vi "WriteHeader.vi"(2 "Filename":string, 3 "NXT":T1={"Hardware"="NXT", "Flattened String"=""}, 8 "File Size (2048)":u32=2048 caption="File Size (256)") -> (0 "NXT":T1={"Hardware"="NXT", "Flattened String"=""})   [LabVIEW 2010, in "Packet Recorder.lvlib"]
uses:
  Packet Recorder.lvlib
  <vilib>/NXT/Subs/LVHSConnector.ctl
  Components/Components.lvlib
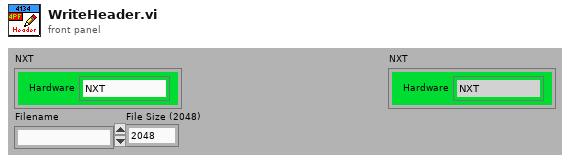
[diagram p1: front panel]
types:
  T1 = typedef "LVHSConnector.ctl" = cluster{"Hardware":string, "Flattened String":string}
  T2 = enum16{"big-endian, network order", "native, host order", "little-endian"}
  T3 = cluster{"1B1-12:2B1-12:1POV:2POV":bool[], "1LXY:RXY:2LXY:RXY":bool[]}
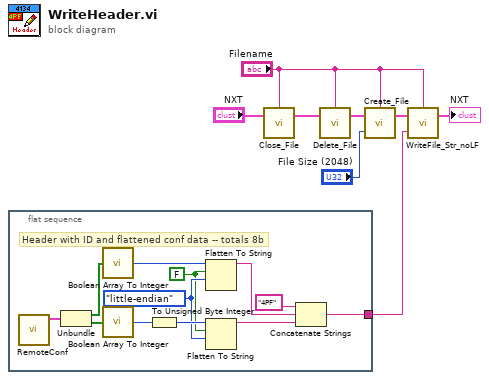
[diagram p0: block diagram]
diagram:
  n1 = flat-sequence {
    tunnel: [w9] -> w8
    frame #0 {
      w14 = T2."little-endian" ("byte order (0:big-endian, network order)")
      w13 = FALSE ("prepend array or string size? (T)")
      # "Header with ID and flattened conf data -- totals 8b"
      n2 = call "RemoteConf.vi"() -> ("Conf"=w20:T3)  [unwired: 11 in]
      n3 = Unbundle(w20) -> ("1B1-12:2B1-12:1POV:2POV"=w18:bool[], "1LXY:RXY:2LXY:RXY"=w19:bool[])
      n4 = call "Boolean Array To Integer.vi"("Boolean array"=w18) -> ("number"=w16:u32)  [unwired: 4 in]
      n5 = call "Boolean Array To Integer.vi"("Boolean array"=w19) -> ("number"=w17:u32)  [unwired: 4 in]
      n6 = To Unsigned Byte Integer(number=w17) -> (unsigned 8bit integer=w15:u8)
      n7 = Flatten To String(anything=w16, prepend array or string size? (T)=w13, byte order (0:big-endian, network order)=w14) -> (data string=w11:string)  [unwired: 1 in, 2 out]
      n8 = Flatten To String(anything=w15, prepend array or string size? (T)=w13, byte order (0:big-endian, network order)=w14) -> (data string=w12:string)  [unwired: 1 in, 2 out]
      n9 = Concatenate Strings("4PF" ("string"), w11, w12) -> (w9:string)
    }
  }
  n10 = call <vilib>:"Close_File.vi"("NXT"="NXT", "Filename"="Filename") -> ("NXT"=w2:T1)  [unwired: 2 in]
  n11 = call <vilib>:"Delete_File.vi"("NXT"=w2, "Filename"="Filename") -> ("NXT"=w5:T1)  [unwired: 2 in]
  n12 = call <vilib>:"Create_File.vi"("File Size (256)"="File Size (2048)", "NXT"=w5, "Filename"="Filename") -> ("NXT"=w6:T1)  [unwired: 1 in]
  n13 = call <vilib>:"WriteFile_Str_noLF.vi"("String"=w8, "NXT"=w6, "Filename"="Filename") -> ("NXT"=→"NXT":T1)  [unwired: 1 in]
